vi "Convert VI Information Array to Table.vi"(11 "VI Information Array":T1[](array[typedef])) -> (3 "Array Out":string[][](array[string]))   [LabVIEW 2019, in "Engine.lvclass"]
uses:
  Engine.lvclass
  VI Information.ctl
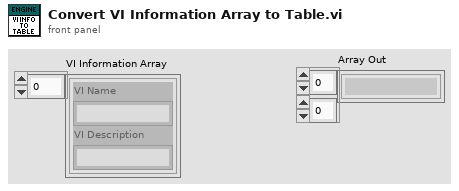
[diagram p1: front panel]
types:
  T1 = typedef "Engine.lvclass/VI Information.ctl" = cluster{"VI Name":string, "VI Description":string}
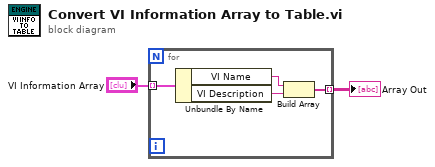
[diagram p0: block diagram]
diagram:
  n1 = for {
    tunnel: "VI Information Array" -> [w6] mode=indexing
    tunnel: [w3] -> w1 mode=indexing
    n2 = Unbundle By Name(w6) -> ("VI Name"=w5:string, "VI Description"=w4:string)
    n3 = Build Array(w5, w4) -> (w3:string[])
  }
  "Array Out" <- w1
